vi "Calibrate Channel.vi"(4 "Ctrl Name":string, 6 "Row":i32, 8 "error in":errorcluster, 9 "Hdr Names":T3[](array[typedef]), 10 "Chassis Name":string, 11 "Strain in":refnum<class "Strain.lvclass">) -> (0 "error out":errorcluster, 2 "Cell Contents":T1[](array[typedef]))   [LabVIEW 2018, in "Measurement Channels.lvlib" / "Strain.lvclass"]
uses:
  Strain.lvclass
  C:/Users/Jeff Tipps/Documents/DAQMan/source/Classes/Measurements/Class Channel/Channel.lvclass
  Common/Controls/HeaderNames.ctl
  SubVIs Table/Custom Ctls Table/ge_CellContents.ctl
  <vilib>/Utility/miscctls.llb/LVPoint32TypeDef.ctl
  Class Channel/Read Device.vi
  Read Lead Res.vi
  <vilib>/DAQmx/configure/timing.llb/DAQmx Timing (Sample Clock).vi
  <vilib>/DAQmx/calibration/calibrationInfo.llb/DAQmx Perform Shunt Calibration Ex (Strain).vi
  <resource>/objmgr/daqmx.rc
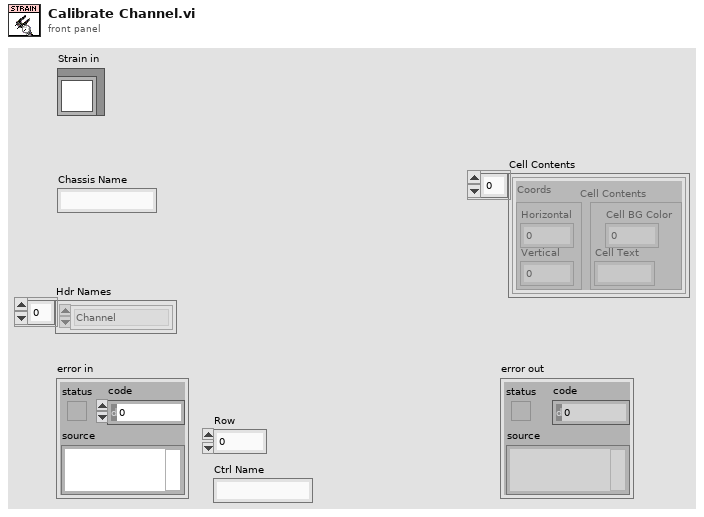
[diagram p1: front panel]
types:
  T1 = typedef "ge_CellContents.ctl" = cluster{"Cell Contents":cluster{"Cell Text":string, "Cell BG Color":u32}, "Coords":T2}
  T2 = typedef "LVPoint32TypeDef.ctl" = cluster{"Horizontal":i32, "Vertical":i32}
  T3 = typedef "HeaderNames.ctl" = enum16{"Channel", "Device", "Spacer", "Description", "MB", "Range", "Terminal", "Coupling", "Thresh (V)", "Pulse/Rev", "Slope", "Min EU", "Min RPM", "mV/EU", "Iex", "Temp Units", "Type", "CJC Src", "CJC Val", "Ro", "Wire Cfg", "Strain Mode", "Vex", "Bridge Type", "GF", "Gauge Res", "Poisson", "Lead Res", "Init Strain", "GAF", "Scale", "Offset", "Unit (EU)", "dB?", "dB Ref", "Cal Mag", "Cal Units", "Max Temp", "Min Temp", "Max Strain", "Min Strain"}
  T4 = cluster{cluster{"Float String":string, "Normal":u32}, cluster{"Row":i32, "index of element":i32}}
  T5 = cluster{cluster{string, "Cell Color":u32}, cluster{"Row":i32, "index of element":i32}}[]
  T6 = cluster{cluster{"Float String":string, "Normal":u32}, cluster{"Row":i32, "index of element":i32}}[]
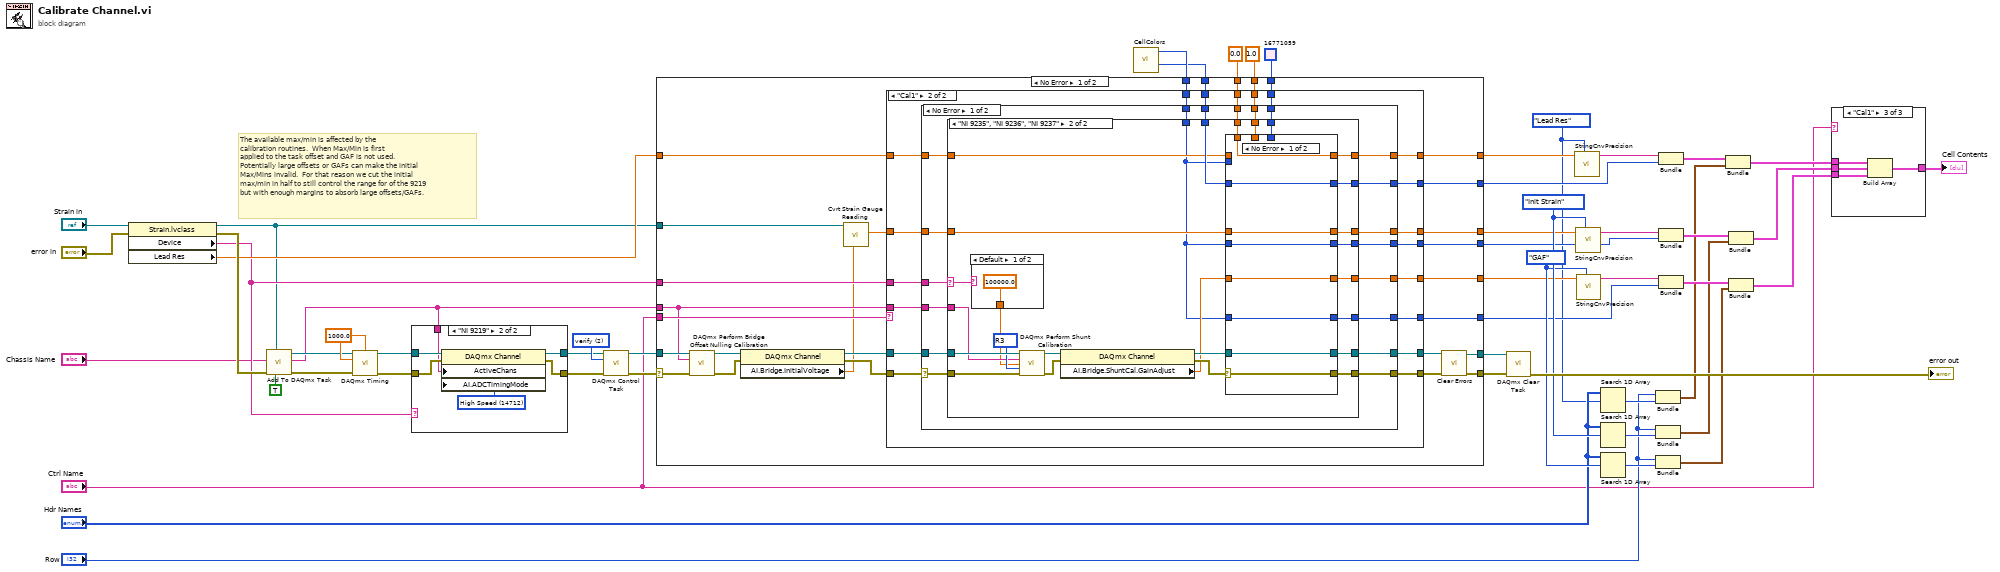
[diagram p0: block diagram]
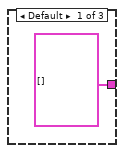
[diagram p2: hidden frame]
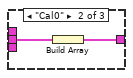
[diagram p3: hidden frame]
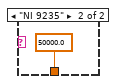
[diagram p8: hidden frame]
diagram:
  w12 = HeaderNames."GAF" ("Header")
  w13 = HeaderNames."Init Strain" ("Header")
  w1 = HeaderNames."Lead Res" ("Header")
  w52 = 2 items=["verify"=2, "reserve"=4, "commit"=3, "unreserve"=5, "abort"=6] ("action")
  w45 = 1000.0 ("rate")
  # "The available max/min is affected by the\ncalibration routines.  When Max/Min is first\napplied to the task offset and GAF is not used.\nPotentially large offsets or GAFs can make the initial\nMax/Mins invalid.  For that reason we cut the initial\nmax/min in half to still control the range for of the 9219\nbut with enough margins to absorb large offsets/GAFs."
  n1 = property class="Strain.lvclass"(reference="Strain in", error in="error in") -> (reference out=w33:refnum<class "Strain.lvclass">, error out=w38:errorcluster, "Device"=w34:string, "Lead Res"=w35:dbl)
  n2 = call-dynamic "Add To DAQmx Task.vi"("Ignore Cal? (F)"=TRUE, "Strain in"=w33, "error in (no error)"=w38, "Chassis Name"="Chassis Name") -> ("error out"=w39:errorcluster, "Phys Chan Added"=w36:string, "task out"=w40:refnum<k21>)  [unwired: 5 in]
  n3 = call-poly <vilib>:"DAQmx Timing.vi"("task/channels in"=w40, "samples per channel"=w45, "rate"=w45, "error in"=w39) -> ("task out"=w44:refnum<k21>, "error out"=w41:errorcluster)  [unwired: 10 in]
  n4 = case shown="\"NI 9219\"" w34 {
    tunnel: w44 -> [w57 w62]
    tunnel: [w57 w61] -> w43
    tunnel: [w56 w60] -> w42
    tunnel: w41 -> [w56 w59]
    tunnel: w36 -> [_ w58]
    frame Default {
    }
    frame "NI 9219" {
      w63 = 14712 items=["High Resolution"=10195, "High Speed"=14712, "Best 50 Hz Rejection"=14713, "Best 60 Hz Rejection"=14714, "Custom"=10137] ("AI.ADCTimingMode")
      n5 = property class="DAQmx Channel"(reference=w62, error in=w59, "ActiveChans"=w58, "AI.ADCTimingMode"=w63) -> (reference out=w61:refnum<k21>, error out=w60:errorcluster)
    }
  }
  n6 = call <vilib>:"DAQmx Control Task.vi"("task/channels in"=w43, "action"=w52, "error in"=w42) -> ("task out"=w53:refnum<k21>, "error out"=w51:errorcluster)  [unwired: 11 in]
  n7 = call "CellColors.vi"() -> ("Coerced"=w46:u32, "Normal"=w48:u32)  [unwired: 8 in, 2 out]
  n8 = case shown="No Error" w51 {
    selector: w51 -> [w68 w219]
    tunnel: [w90 w218] -> w55
    tunnel: [w77 w219] -> w54
    tunnel: [w89 w216] -> w9
    tunnel: w53 -> [w69 w218]
    tunnel: [w85 w217] -> w7
    tunnel: sgl 0.0 -> [w83 w217]
    tunnel: 1.0 ("AI.Bridge.ShuntCal.GainAdjust") -> [w82 w216]
    tunnel: [w81 w215] -> w6
    tunnel: [w80 w215] -> w8
    tunnel: w48 -> [w79 w213]
    tunnel: u32 16771059 -> [w78 w215]
    tunnel: w34 -> [w75 _]
    tunnel: w46 -> [w74 _]
    tunnel: "Ctrl Name" -> [w73 _]
    tunnel: w35 -> [w72 w214]
    tunnel: [w71 w214] -> w11
    tunnel: [w70 w213] -> w10
    tunnel: w36 -> [w67 _]
    tunnel: w33 -> [w64 _]
    frame No Error {
      n9 = call <vilib>:"DAQmx Perform Bridge Offset Nulling Calibration.vi"("task/channels in"=w69, "channels"=w67, "error in"=w68) -> ("task out"=w88:refnum<k21>, "error out"=w87:errorcluster)  [unwired: 11 in]
      n10 = property class="DAQmx Channel"(reference=w88, error in=w87) -> (reference out=w86:refnum<k21>, error out=w84:errorcluster, "AI.Bridge.InitialVoltage"=w66:dbl)
      n11 = call "Cvrt Strain Gauge Reading.vi"("Vinit (0.0)"=w66, "Strain in"=w64) -> ("Strain"=w65:sgl)  [unwired: 9 in]
      n12 = case shown="\"Cal1\"" w73 {
        tunnel: [w102 w135] -> w90
        tunnel: [w97 w134] -> w89
        tunnel: w86 -> [w101 w133]
        tunnel: [w94 w132] -> w85
        tunnel: w65 -> [w93 w131]
        tunnel: w84 -> [w104 w130]
        tunnel: w83 -> [w95 w129]
        tunnel: w82 -> [w96 w128]
        tunnel: [w100 w127] -> w81
        tunnel: [w99 w126] -> w80
        tunnel: w79 -> [w91 w125]
        tunnel: w78 -> [w98 w124]
        tunnel: [w103 w123] -> w76
        tunnel: w75 -> [_ w122]
        tunnel: w74 -> [_ w121]
        tunnel: w72 -> [w92 w120]
        tunnel: [w92 w119] -> w71
        tunnel: [w91 w118] -> w70
        tunnel: w67 -> [_ w117]
        frame "Cal0", Default {
          n13 = case shown="No Error" w104 {
            selector: w104 -> [w110 w113]
            tunnel: [w110 w113] -> w103
            tunnel: w101 -> [w109 w114]
            tunnel: [w109 w114] -> w102
            tunnel: w91 -> [w108 _]
            tunnel: [w108 w115] -> w100
            tunnel: w91 -> [w107 w116]
            tunnel: [w107 w116] -> w99
            tunnel: w98 -> [_ w115]
            tunnel: w96 -> [w105 w112]
            tunnel: [w105 w112] -> w97
            tunnel: [w106 w111] -> w94
            tunnel: w95 -> [_ w111]
            tunnel: w93 -> [w106 _]
            frame No Error {
            }
            frame Error {
            }
          }
        }
        frame "Cal1" {
          n14 = case shown="No Error" w130 {
            selector: w130 -> [w153 w209]
            tunnel: [w151 w210] -> w135
            tunnel: [w152 w209] -> w123
            tunnel: [w147 w211] -> w134
            tunnel: w133 -> [w154 w210]
            tunnel: [w143 w212] -> w132
            tunnel: w131 -> [w144 _]
            tunnel: w129 -> [w137 w212]
            tunnel: w128 -> [w146 w211]
            tunnel: [w150 w208] -> w127
            tunnel: [w149 w208] -> w126
            tunnel: w125 -> [w148 w206]
            tunnel: w124 -> [w145 w208]
            tunnel: w122 -> [w142 _]
            tunnel: w121 -> [w141 _]
            tunnel: w120 -> [w140 w207]
            tunnel: [w139 w207] -> w119
            tunnel: [w138 w206] -> w118
            tunnel: w117 -> [w136 _]
            frame No Error {
              n15 = case shown="\"NI 9235\", \"NI 9236\", \"NI 9237\"" w142 {
                selector: w142 -> [_ w163]
                tunnel: w154 -> [w158 w185]
                tunnel: w153 -> [w157 w184]
                tunnel: [w157 w182] -> w152
                tunnel: [w158 w180] -> w151
                tunnel: [w155 w179] -> w150
                tunnel: [w159 w178] -> w149
                tunnel: w148 -> [w155 w165]
                tunnel: [w160 w177] -> w147
                tunnel: w146 -> [w160 w175]
                tunnel: w145 -> [_ w174]
                tunnel: w144 -> [w161 w172]
                tunnel: [w161 w171] -> w143
                tunnel: w141 -> [w159 w167]
                tunnel: w140 -> [w156 w166]
                tunnel: [w156 w169] -> w139
                tunnel: [w155 w168] -> w138
                tunnel: w137 -> [_ w170]
                tunnel: w136 -> [_ w164]
                frame Default {
                }
                frame "NI 9235", "NI 9236", "NI 9237" {
                  w173 = 12467 items=["R1"=12465, "R2"=12466, "R3"=12467, "R4"=14813] ("shunt element location")
                  n16 = case shown="Default" w163 {
                    tunnel: [100000.0 ("shunt resistance") 50000.0 ("shunt resistance")] -> w162
                    frame Default {
                    }
                    frame "NI 9235" {
                    }
                  }
                  n17 = call-poly <vilib>:"DAQmx Perform Shunt Calibration.vi"("task/channels in"=w185, "channels"=w164, "shunt resistance"=w162, "shunt element location"=w173, "error in"=w184) -> ("task out"=w186:refnum<k21>, "error out"=w187:errorcluster)  [unwired: 9 in]
                  n18 = property class="DAQmx Channel"(reference=w186, error in=w187) -> (reference out=w181:refnum<k21>, error out=w183:errorcluster, "AI.Bridge.ShuntCal.GainAdjust"=w176:dbl)
                  n19 = case shown="No Error" w183 {
                    selector: w183 -> [w197 w201]
                    tunnel: [w197 w201] -> w182
                    tunnel: [w196 w202] -> w180
                    tunnel: w181 -> [w196 w202]
                    tunnel: w165 -> [w195 w205]
                    tunnel: [w195 w205] -> w179
                    tunnel: w165 -> [w194 _]
                    tunnel: [w194 w203] -> w178
                    tunnel: w176 -> [w193 _]
                    tunnel: [w193 w204] -> w177
                    tunnel: w175 -> [_ w204]
                    tunnel: w174 -> [_ w203]
                    tunnel: [w192 w200] -> w171
                    tunnel: w172 -> [w192 w200]
                    tunnel: w170 -> [w191 _]
                    tunnel: [w191 w199] -> w169
                    tunnel: w167 -> [w190 _]
                    tunnel: [w190 w198] -> w168
                    tunnel: w166 -> [_ w199]
                    tunnel: w165 -> [_ w198]
                    frame No Error {
                    }
                    frame Error {
                    }
                  }
                }
              }
            }
            frame Error {
            }
          }
        }
      }
      n20 = call <vilib>:"Clear Errors.vi"("error in (no error)"=w76) -> ("error out"=w77:errorcluster)  [unwired: 5 in, 1 out]
    }
    frame Error {
    }
  }
  n21 = call <vilib>:"DAQmx Clear Task.vi"("task in"=w55, "error in"=w54) -> ("error out"=→"error out":errorcluster)  [unwired: 13 in]
  n22 = call "StringCnvPrecision.vi"("Number"=w11, "Header"=w1) -> ("Float String"=w16:string)  [unwired: 5 in]
  n23 = call "StringCnvPrecision.vi"("Number"=w7, "Header"=w13) -> ("Float String"=w15:string)  [unwired: 5 in]
  n24 = call "StringCnvPrecision.vi"("Number"=w9, "Header"=w12) -> ("Float String"=w14:string)  [unwired: 5 in]
  n25 = Search 1D Array(1D array="Hdr Names", element=w1) -> (index of element=w22:i32)  [unwired: 1 in]
  n26 = Search 1D Array(1D array="Hdr Names", element=w13) -> (index of element=w28:i32)  [unwired: 1 in]
  n27 = Search 1D Array(1D array="Hdr Names", element=w12) -> (index of element=w27:i32)  [unwired: 1 in]
  n28 = Bundle("Row"="Row", "index of element"=w22) -> (w20:cluster{"Row":i32, "index of element":i32})  [unwired: 1 in]
  n29 = Bundle("Row"="Row", "index of element"=w28) -> (w19:cluster{"Row":i32, "index of element":i32})  [unwired: 1 in]
  n30 = Bundle("Row"="Row", "index of element"=w27) -> (w18:cluster{"Row":i32, "index of element":i32})  [unwired: 1 in]
  n31 = Bundle("Float String"=w16, "Normal"=w10) -> (w26:cluster{"Float String":string, "Normal":u32})  [unwired: 1 in]
  n32 = Bundle("Float String"=w15, "Normal"=w6) -> (w25:cluster{"Float String":string, "Normal":u32})  [unwired: 1 in]
  n33 = Bundle("Float String"=w14, "Normal"=w8) -> (w21:cluster{"Float String":string, "Normal":u32})  [unwired: 1 in]
  n34 = Bundle(w26, w20) -> (w24:T4)  [unwired: 1 in]
  n35 = Bundle(w25, w19) -> (w23:T4)  [unwired: 1 in]
  n36 = Bundle(w21, w18) -> (w17:T4)  [unwired: 1 in]
  n37 = case shown="\"Cal1\"" "Ctrl Name" {
    tunnel: [T5 [] w222 w226] -> w2
    tunnel: w24 -> [_ _ w225]
    tunnel: w23 -> [_ w221 w224]
    tunnel: w17 -> [_ _ w223]
    frame Default {
    }
    frame "Cal0" {
      n38 = Build Array(w221) -> (w222:T6)
    }
    frame "Cal1" {
      n39 = Build Array(w225, w224, w223) -> (w226:T6)
    }
  }
  "Cell Contents" <- w2
